vi "Cast To Variant (Array).vi"(8 "error in (no error)":errorcluster, 9 "datatype and defaults":variant, 11 "JSON Value in":refnum<class "JSON Value.lvclass">) -> (0 "error out":errorcluster, 2 "Variant":variant)   [LabVIEW 2016, in "JSON Value.lvclass"]
doc: "Populates a variant with the data contained in the given JSON instance. Valid types for datatype and defaults are: string, boolean, double, and a cluster of named controls of strings, booleans, doubles, or nested clusters.\n\nIf a given cluster contains values that aren't present in the JSON Object instance, the value in the datatype and defaults control is used instead and the defaulted keys output will contain the name of the path in the cluster to the control."
uses:
  JSON Value.lvclass
  Array/Index Array/Index Array (JSON).vi
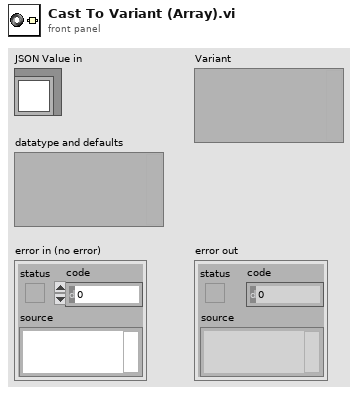
[diagram p1: front panel]
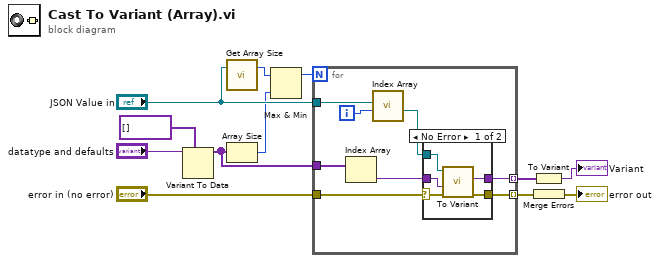
[diagram p0: block diagram]
diagram:
  n1 = Variant To Data(type=variant[] [], Variant="datatype and defaults") -> (data=w4:variant[])  [unwired: 1 in, 1 out]
  n2 = call "Get Array Size.vi"("JSON Value in"="JSON Value in") -> ("size(s)"=w2:i32)  [unwired: 1 in, 1 out]
  n3 = Array Size(array=w4) -> (size(s)=w3:i32)
  n4 = Max & Min(x=w2, y=w3) -> (max(x,y)=w1:i32)  [unwired: 1 out]
  n5 = for {
    N: w1 -> [_]
    tunnel: w4 -> [w15]
    tunnel: "JSON Value in" -> [w20]
    tunnel: [w19] -> w9 mode=indexing
    tunnel: [w18] -> w7 mode=indexing
    tunnel: "error in (no error)" -> [w17]
    i -> [w16]
    n6 = Index Array(array=w15) -> (element=w13:variant)  [unwired: 1 in]
    n7 = call-poly "Index Array.vi"("index"=w16, "JSON Value in"=w20) -> ("JSON Value out"=w14:refnum<class "JSON Value.lvclass">)  [unwired: 8 in, 1 out]
    n8 = case shown="No Error" w17 {
      selector: w17 -> [w21 w27]
      tunnel: w14 -> [w23 _]
      tunnel: [w24 w26] -> w19
      tunnel: [w22 w27] -> w18
      tunnel: w13 -> [w25 w26]
      frame No Error {
        n9 = call "To Variant.vi"("error in (no error)"=w21, "datatype and defaults"=w25, "JSON Value in"=w23) -> ("error out"=w22:errorcluster, "Variant"=w24:variant)  [unwired: 6 in, 1 out]
      }
      frame Error {
      }
    }
  }
  n10 = To Variant(anything=w9) -> (Variant=→"Variant":variant)
  n11 = Merge Errors(w7) -> (→"error out":errorcluster)
